vi "Uniqe number.vi"() -> (6 "Uniqe 64u number":u64, 10 "Uniqe 32u number":u32)   [LabVIEW 2010]
doc: "Supplyes a new uniqe number each time called."
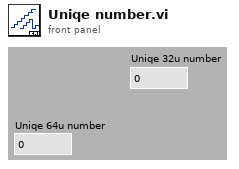
[diagram p1: front panel]
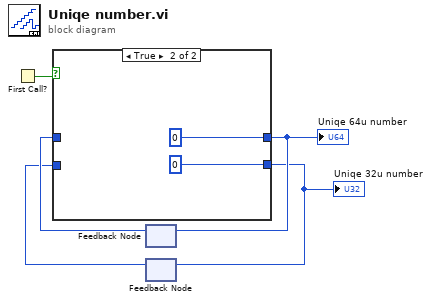
[diagram p0: block diagram]
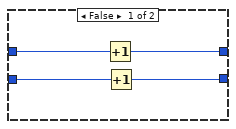
[diagram p2: hidden frame]
diagram:
  n1 = First Call?() -> (First Call?: T/F=w3:bool)
  n2 = feedback #1() -> (w5:u64)  [unwired: 1 in]
  n3 = feedback #2() -> (w1:u32)  [unwired: 1 in]
  n4 = case shown="True" w3 {
    tunnel: [w8 u64 0] -> w4
    tunnel: w5 -> [w9 _]
    tunnel: [w7 u32 0] -> w2
    tunnel: w1 -> [w6 _]
    frame False {
      n5 = Increment(x=w9) -> (x+1=w8:u64)
      n6 = Increment(x=w6) -> (x+1=w7:u32)
    }
    frame True {
    }
  }
  "Uniqe 64u number" <- w4
  "Uniqe 32u number" <- w2
  n7 = feedback-in #1(w4) -> ()
  n8 = feedback-in #2(w2) -> ()
